vi "browseVariantArray.vi"(4 "Array of Variants":variant[](array[variant]), 6 "error in":errorcluster, 7 "ParentTag":string, 9 "VariantProbe.lvclass in":refnum<class "Failures_VariantTree__VP.lvclass">) -> (0 "error out":errorcluster, 3 "VariantProbe.lvclass out":refnum<class "Failures_VariantTree__VP.lvclass">)   [LabVIEW 2013, in "Failures_VariantTree__VP.lvclass"]
uses:
  Failures_VariantTree__VP.lvclass
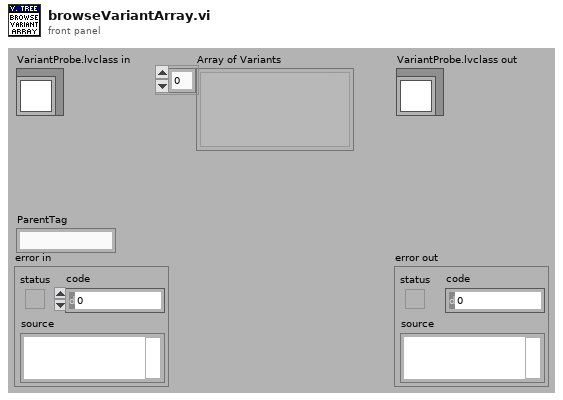
[diagram p1: front panel]
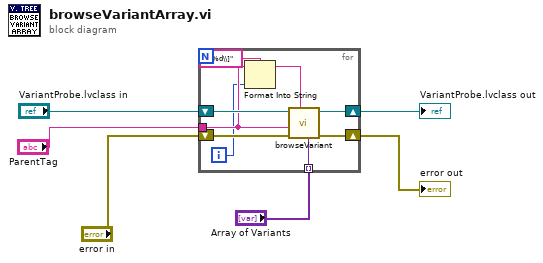
[diagram p0: block diagram]
diagram:
  n1 = for {
    tunnel: "ParentTag" -> [w10]
    shift-right: [w15] -> w4
    shift-left: "VariantProbe.lvclass in" -> [w12]
    tunnel: "Array of Variants" -> [w14] mode=indexing
    shift-right: [w13] -> w5
    shift-left: "error in" -> [w11]
    i -> [w9]
    n2 = Format Into String(format string="\\[%d\\]", initial string=w10, w9) -> (resulting string=w7:string)  [unwired: 1 in, 1 out]
    n3 = call-dynamic "browseVariant.vi"("Variant"=w14, "Name"=w7, "error in (no error)"=w11, "ParentTag"=w10, "VariantProbe.lvclass in"=w12) -> ("error out"=w13:errorcluster, "VariantProbe.lvclass out"=w15:refnum<class "Failures_VariantTree__VP.lvclass">)  [unwired: 3 in]
  }
  "error out" <- w5
  "VariantProbe.lvclass out" <- w4
